vi "Variant to String.vi"(8 "error in (no error)":errorcluster, 10 "Variant":variant, 11 "String Value in":refnum<class "String Value.lvclass">) -> (0 "error out":errorcluster, 2 "String":string, 3 "String Value out":refnum<class "String Value.lvclass">)   [LabVIEW 2020, in "Composed Columns.lvlib" / "String Value.lvclass"]
uses:
  String Value.lvclass
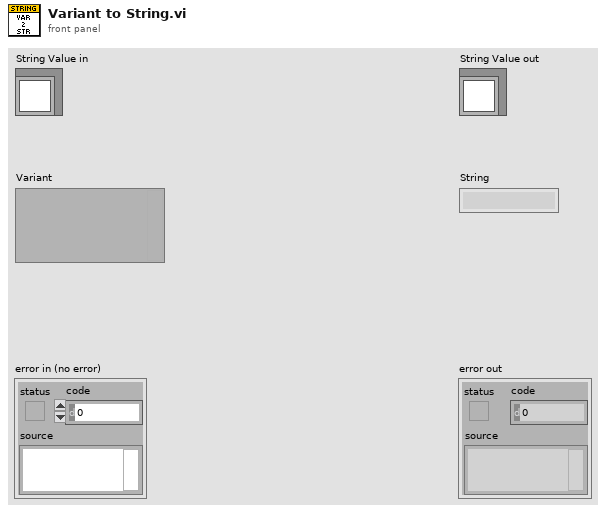
[diagram p1: front panel]
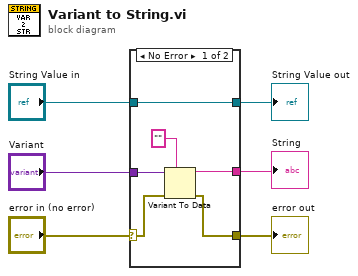
[diagram p0: block diagram]
diagram:
  n1 = case shown="No Error" "error in (no error)" {
    selector: "error in (no error)" -> [w8 w13]
    tunnel: "String Value in" -> [w12 w14]
    tunnel: [w12 w14] -> w4
    tunnel: [w7 w13] -> w3
    tunnel: "Variant" -> [w11 _]
    tunnel: [w9 _] -> w1
    frame No Error {
      n2 = Variant To Data(error in=w8, type="" ("String"), Variant=w11) -> (data=w9:string, error out=w7:errorcluster)
    }
    frame Error {
    }
  }
  "error out" <- w3
  "String Value out" <- w4
  "String" <- w1
